vi "SQL查询.vi"(7 "condition":string, 9 "columns":string[](array[string]), 10 "table输入":string(combo), 11 "database":string(combo)) -> (0 "error out":errorcluster, 2 "columns输出":string[](array[string]), 3 "data":string[][](table))   [LabVIEW 2016, in "数据传输系统.lvlib"]
uses:
  <vilib>/Utility/sysdir.llb/System Directory Type.ctl
  <vilib>/addons/database/Connection.llb/DB Tools Open Connec (String).vi
  <vilib>/addons/database/_DB Variant To Data/Database Variant To Data.xnode
  <vilib>/addons/database/NI_Database_API.lvlib
panel:
  out "元素":string
  out "子数组":string[](array[string])
  in  "error in (no error)":errorcluster
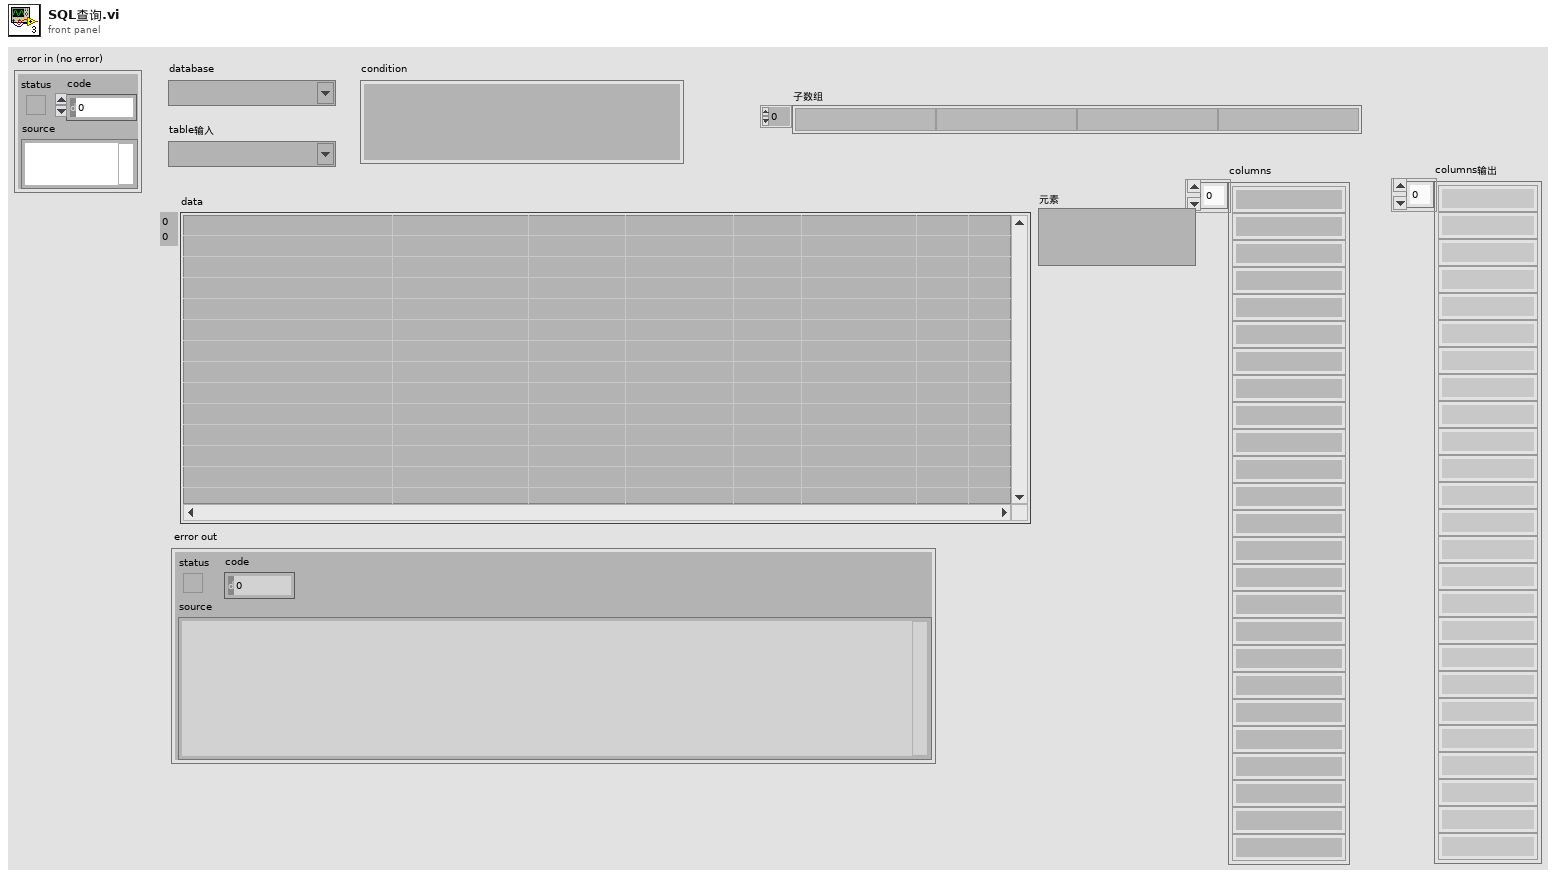
[diagram p1: front panel]
types:
  T1 = typedef "System Directory Type.ctl" = i32
  T2 = typedef "NI_Database_API.lvlib/Conn ObjectReference.ctl" = refnum<k1>
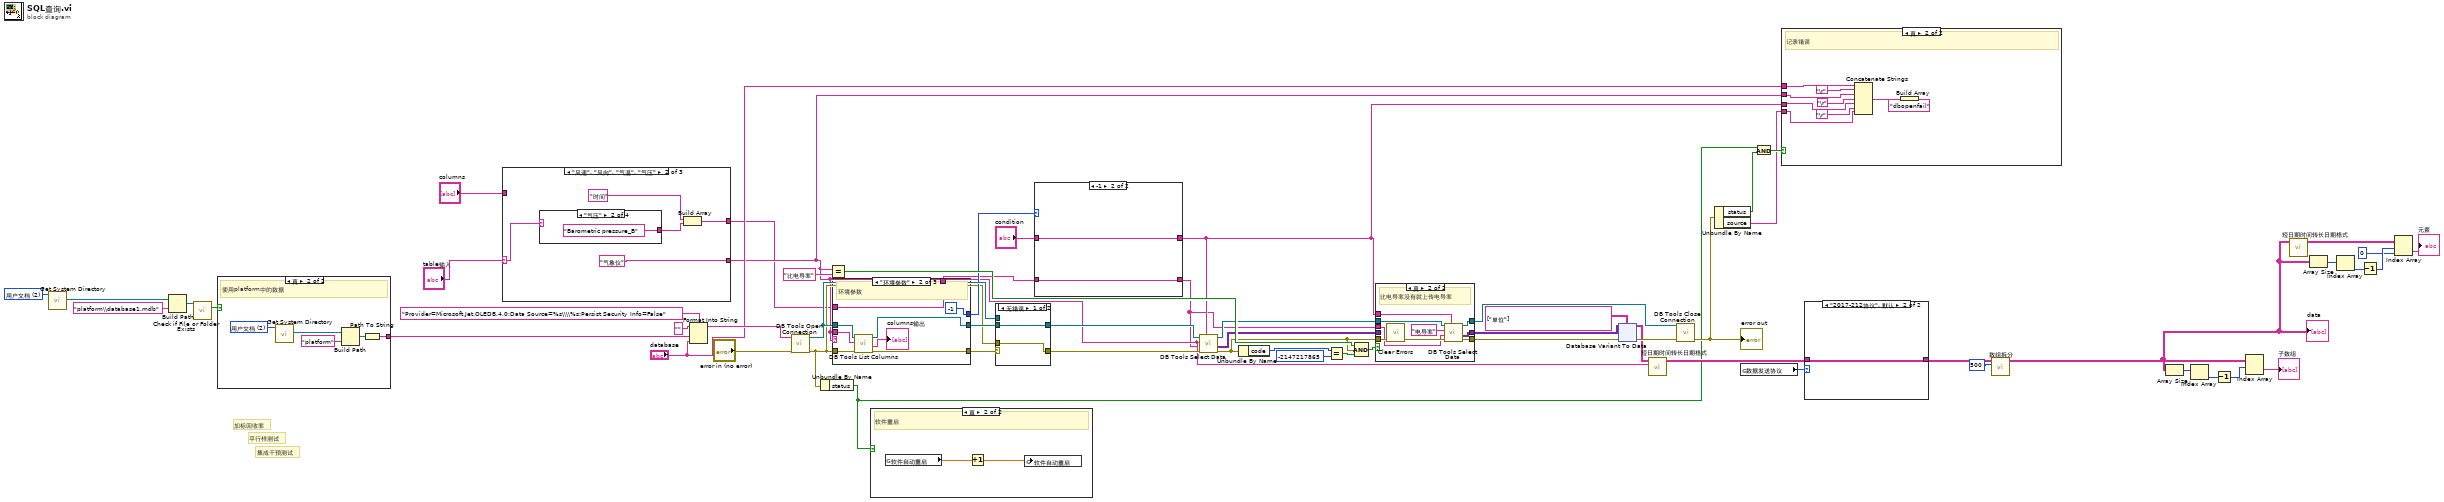
[diagram p0: block diagram]
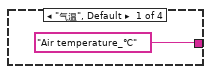
[diagram p5: hidden frame]
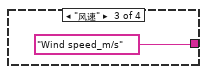
[diagram p6: hidden frame]
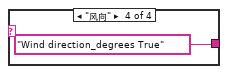
[diagram p7: hidden frame]
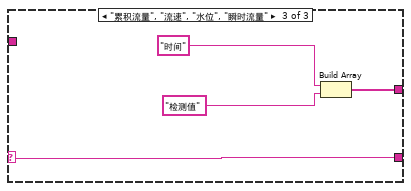
[diagram p8: hidden frame]
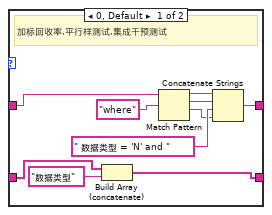
[diagram p9: hidden frame]
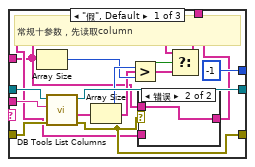
[diagram p11: hidden frame]
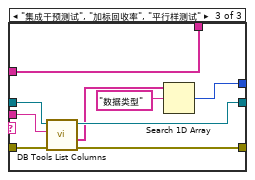
[diagram p13: hidden frame]
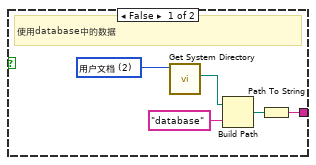
[diagram p15: hidden frame]
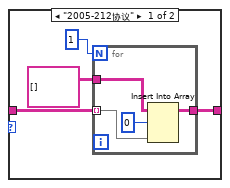
[diagram p16: hidden frame]
diagram:
  w47 = T1 2 items=["用户目录"=0, "用户桌面"=1, "用户文档"=2, "用户应用程序数据"=3, "用户设置"=4, "用户临时目录"=5, "公共文档"=6, "公共应用程序数据"=7, "公共设置"=8, "公共缓存"=13, "系统核心库"=9, "系统安装库"=10, "应用程序文件"=11, "启动盘根目录"=12] ("system directory type")
  # "集成干预测试"
  # "平行样测试"
  # "加标回收率"
  n1 = call <vilib>:"Get System Directory.vi"("system directory type"=w47) -> ("system directory"=w48:path)  [unwired: 10 in]
  n2 = Build Path(base path=w48, name or relative path="platform\\database1.mdb" ("condition")) -> (appended path=w46:path)
  n3 = call <vilib>:"Check if File or Folder Exists.vi"("path"=w46) -> ("file or folder exists?"=w44:bool)  [unwired: 8 in, 2 out]
  n4 = case shown="真" w44 {
    tunnel: [w62 w67] -> w43
    frame False {
      w65 = T1 2 items=["用户目录"=0, "用户桌面"=1, "用户文档"=2, "用户应用程序数据"=3, "用户设置"=4, "用户临时目录"=5, "公共文档"=6, "公共应用程序数据"=7, "公共设置"=8, "公共缓存"=13, "系统核心库"=9, "系统安装库"=10, "应用程序文件"=11, "启动盘根目录"=12] ("system directory type")
      # "使用database中的数据"
      n5 = call <vilib>:"Get System Directory.vi"("system directory type"=w65) -> ("system directory"=w64:path)  [unwired: 10 in]
      n6 = Build Path(base path=w64, name or relative path="database" ("condition")) -> (appended path=w66:path)
      n7 = Path To String(path=w66) -> (string=w62:string)
    }
    frame True {
      w71 = T1 2 items=["用户目录"=0, "用户桌面"=1, "用户文档"=2, "用户应用程序数据"=3, "用户设置"=4, "用户临时目录"=5, "公共文档"=6, "公共应用程序数据"=7, "公共设置"=8, "公共缓存"=13, "系统核心库"=9, "系统安装库"=10, "应用程序文件"=11, "启动盘根目录"=12] ("system directory type")
      # "使用platform中的数据"
      n8 = call <vilib>:"Get System Directory.vi"("system directory type"=w71) -> ("system directory"=w70:path)  [unwired: 10 in]
      n9 = Build Path(base path=w70, name or relative path="platform" ("condition")) -> (appended path=w68:path)
      n10 = Path To String(path=w68) -> (string=w67:string)
    }
  }
  n11 = case shown="\"风速\", \"风向\", \"气温\", \"气压\"" "table输入" {
    selector: "table输入" -> [w73 w77 w83]
    tunnel: [w73 "气象仪" w83] -> w9
    tunnel: "columns" -> [w72 _ _]
    tunnel: [w72 w74 w85] -> w2
    frame "", Default {
    }
    frame "风速", "风向", "气温", "气压" {
      n12 = case shown="\"气压\"" w77 {
        tunnel: ["Air temperature_℃" "Barometric pressure_B" "Wind speed_m/s" "Wind direction_degrees True"] -> w75
        frame "气温", Default {
        }
        frame "气压" {
        }
        frame "风速" {
        }
        frame "风向" {
        }
      }
      n13 = Build Array("时间", w75) -> (w74:string[])
    }
    frame "累积流量", "流速", "水位", "瞬时流量" {
      n14 = Build Array("时间", "检测值") -> (w85:string[])
    }
  }
  n15 = Format Into String(format string="Provider=Microsoft.Jet.OLEDB.4.0;Data Source=%s\\\\%s;Persist Security Info=False" ("格式字符串"), initial string="" ("初始字符串"), w43, "database") -> (resulting string=w56:string)  [unwired: 1 in, 1 out]
  n16 = call-poly <vilib>:"DB Tools Open Connection.vi"("error in (no error)"="error in (no error)", "connection information"=w56) -> ("error out"=w15:errorcluster, "connection reference"=w27:T2)  [unwired: 6 in]
  n17 = Unbundle By Name(w15) -> ("status"=w12:bool)
  n18 = Equal?(x=w9, y="比电导率") -> (x = y?=w41:bool)
  n19 = case shown="\"环境参数\"" w9 {
    tunnel: w27 -> [w98 w109 w118]
    tunnel: w15 -> [w95 w108 w116]
    tunnel: [w96 w107 w115] -> w29
    tunnel: [w90 w106 w114] -> w30
    tunnel: w9 -> [w97 w105 w117]
    tunnel: [-1 ("index of element") -1 ("index of element") w111] -> w25
    tunnel: w2 -> [w87 w102 w110]
    tunnel: [w88 w102 w110] -> w22
    frame "假", Default {
      # "常规十参数，先读取column"
      n20 = Array Size(array=w87) -> (size(s)=w92:i32)
      n21 = call <vilib>:"DB Tools List Columns.vi"("error in (no error)"=w95, "table"=w97, "connection reference"=w98) -> ("error out"=w90:errorcluster, "columns"=w91:string[], "connection reference out"=w96:T2)  [unwired: 1 in, 1 out]
      n22 = Array Size(array=w91) -> (size(s)=w93:i32)
      n23 = Greater?(x=w93, y=w92) -> (0:w94:bool)
      n24 = Select(t=w87, s=w94, f=w91) -> (s? t:f=w89:string[])
      n25 = case shown="错误" w90 {
        tunnel: w89 -> [w100 _]
        tunnel: [w100 w101] -> w88
        tunnel: w87 -> [_ w101]
        frame No Error {
        }
        frame Error {
        }
      }
    }
    frame "环境参数" {
      # "环境参数"
      n26 = call <vilib>:"DB Tools List Columns.vi"("error in (no error)"=w108, "table"=w105, "connection reference"=w109) -> ("error out"=w106:errorcluster, "columns"=→"columns输出":string[], "connection reference out"=w107:T2)  [unwired: 1 in, 1 out]
    }
    frame "集成干预测试", "加标回收率", "平行样测试" {
      n27 = call <vilib>:"DB Tools List Columns.vi"("error in (no error)"=w116, "table"=w117, "connection reference"=w118) -> ("error out"=w114:errorcluster, "columns"=w113:string[], "connection reference out"=w115:T2)  [unwired: 1 in, 1 out]
      n28 = Search 1D Array(1D array=w113, element="数据类型" ("元素")) -> (index of element=w111:i32)  [unwired: 1 in]
    }
  }
  n29 = case shown="真" w12 {
    frame False {
    }
    frame True {
      # "软件重启"
      n30 = global read "全局1.vi" "软件自动重启"() -> (w120:dbl)
      n31 = Increment(x=w120) -> (x+1=w119:dbl)
      n32 = global write "全局1.vi" "软件自动重启"(w119) -> ()
    }
  }
  n33 = case shown="无错误" w30 {
    selector: w30 -> [_ w124]
    tunnel: w29 -> [w122 _]
    tunnel: [w122 w123] -> w28
    tunnel: w27 -> [_ w123]
    tunnel: [w121 w124] -> w26
    tunnel: w15 -> [w121 _]
    frame No Error {
    }
    frame Error {
    }
  }
  n34 = case "条件结构" shown="-1" w25 {
    tunnel: "condition" -> [w132 w135]
    tunnel: w22 -> [w134 w136]
    tunnel: [w126 w136] -> w1
    tunnel: [w125 w135] -> w8
    frame 0, Default {
      # "加标回收率,平行样测试,集成干预测试"
      n35 = Build Array (concatenate)(w134, "数据类型" ("元素")) -> (w126:string[])
      n36 = Match Pattern(string=w132, regular expression="where" ("正则表达式")) -> (before substring=w130:string, match substring=w129:string, after substring=w127:string)  [unwired: 1 in, 1 out]
      n37 = Concatenate Strings(w130, w129, " 数据类型 = 'N' and " ("字符串"), w127) -> (w125:string)
    }
    frame -1 {
    }
  }
  n38 = call <vilib>:"DB Tools Select Data.vi"("condition"=w8, "error in (no error)"=w26, "columns"=w1, "table"=w9, "connection reference"=w28) -> ("error out"=w34:errorcluster, "data"=w36:variant[][], "connection reference out"=w39:T2)  [unwired: 1 in]
  n39 = Unbundle By Name(w34) -> ("code"=w33:i32)
  n40 = Equal?(x=w33, y=-2147217865 ("code")) -> (x = y?=w31:bool)
  n41 = Compound Arithmetic op=AND ("复合运算")(w41, w34, w31) -> (w40:bool)
  n42 = case shown="真" w40 {
    tunnel: w8 -> [_ w148]
    tunnel: w39 -> [w139 w147]
    tunnel: [w139 w142] -> w38
    tunnel: [w138 w143] -> w37
    tunnel: w36 -> [w138 _]
    tunnel: w34 -> [w137 w145]
    tunnel: [w137 w141] -> w35
    tunnel: w1 -> [_ w140]
    frame False {
    }
    frame True {
      # "比电导率没有就上传电导率"
      n43 = call <vilib>:"Clear Errors.vi"("error in (no error)"=w145) -> ("error out"=w144:errorcluster)  [unwired: 5 in, 1 out]
      n44 = call <vilib>:"DB Tools Select Data.vi"("condition"=w148, "error in (no error)"=w144, "columns"=w140, "table"="电导率", "connection reference"=w147) -> ("error out"=w141:errorcluster, "data"=w143:variant[][], "connection reference out"=w142:T2)  [unwired: 1 in]
    }
  }
  n45 = xnode "Database Variant To Data"("database variant"=w37, "error in (no error)"=w35, "type"=string[][] [["单位"]]) -> ("data"=w55:string[][], "error out"=w58:errorcluster)
  n46 = call "短日期时间转长日期格式.vi"("table输入"=w9, "data"=w55) -> ("输出数组"=w54:string[][])  [unwired: 9 in]
  n47 = call <vilib>:"DB Tools Close Connection.vi"("error in (no error)"=w58, "connection reference"=w38) -> ("error out"=w14:errorcluster)  [unwired: 5 in]
  "error out" <- w14
  n48 = Unbundle By Name(w14) -> ("status"=w13:bool, "source"=w7:string)
  n49 = global read "断电保存全局.vi" "数据发送协议"() -> (w53:enum16{"2005-212协议", "2017-212协议"})
  n50 = And(x=w12, y=w13) -> (x .and. y?=w11:bool)
  n51 = case shown="真" w11 {
    tunnel: "database" -> [_ w156]
    tunnel: w9 -> [_ w154]
    tunnel: w8 -> [_ w152]
    tunnel: w7 -> [_ w150]
    frame False {
    }
    frame True {
      (unwired) "dbopenfail" ("字符串")
      # "记录错误"
      n52 = Concatenate Strings(w156, "\r", w154, "\r", w152, "\r", w150) -> (w149:string)
      n53 = Build Array(w149) -> ()  [unwired: 1 out]
    }
  }
  n54 = case shown="\"2017-212协议\", 默认" w53 {
    tunnel: w54 -> [w158 w165]
    tunnel: [w157 w165] -> w5
    frame "2005-212协议" {
      n55 = for {
        N: 1 -> [_]
        tunnel: string[][] [] ("data") -> [w164]
        tunnel: w158 -> [w163] mode=indexing
        tunnel: [w161] -> w157
        n56 = Insert Into Array(array=w164, index (row)=0 ("索引 (行)"), new element=w163) -> (w161:string[][])  [unwired: 1 in]
      }
    }
    frame "2017-212协议", Default {
    }
  }
  n57 = call "数组拆分.vi"("拆分大小"=500, "输入数据"=w5) -> ("输出数组"=w4:string[][])  [unwired: 9 in]
  "data" <- w4
  n58 = Array Size(array=w4) -> (size(s)=w52:i32[])
  n59 = Index Array(array=w52) -> (element=w50:i32)  [unwired: 1 in]
  n60 = Decrement(x=w50) -> (x-1=w49:i32)
  n61 = Index Array(array=w4, index (row)=w49) -> (element=→"子数组":string[])  [unwired: 1 in]
  n62 = call "短日期时间转长日期格式.vi"("data"=w4) -> ("输出数组"=w21:string[][])  [unwired: 10 in]
  n63 = Array Size(array=w4) -> (size(s)=w20:i32[])
  n64 = Index Array(array=w20) -> (element=w19:i32)  [unwired: 1 in]
  n65 = Decrement(x=w19) -> (x-1=w18:i32)
  n66 = Index Array(array=w21, index (row)=w18, index (col)=0 ("禁用的索引 (列)")) -> (element=→"元素":string)
